vi "ReadCurrent.vi"(8 "error in (no error)":errorcluster, 11 "reference in":refnum<class "VdPhilipsMM-456.lvclass">) -> (0 "error out":errorcluster, 2 "Current":dbl, 3 "reference out":refnum<class "VdPhilipsMM-456.lvclass">)   [LabVIEW 2020, in "MulitMeters.lvlib" / "VdPhilipsMM-456.lvclass"]
uses:
  VdPhilipsMM-456.lvclass
  VdPhilipsMM-456.lvclass/VdPhilipsMM-456.ctl
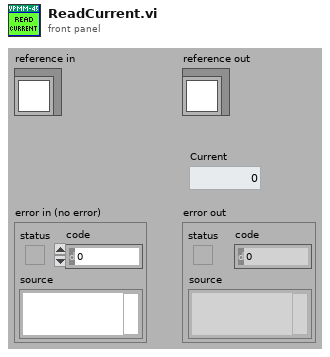
[diagram p1: front panel]
types:
  T1 = typedef "MulitMeters.lvlib/VdPhilipsMM-456.lvclass/ObjectAttributes.ctl" = cluster{"VISA Ref":refnum<visa-resource-name>}
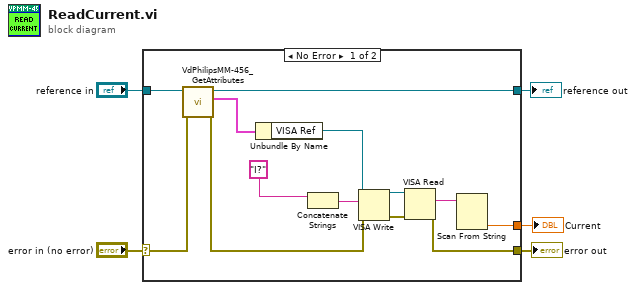
[diagram p0: block diagram]
diagram:
  n1 = case shown="No Error" "error in (no error)" {
    selector: "error in (no error)" -> [w18 w20]
    tunnel: [w9 w20] -> w4
    tunnel: [w15 w19] -> w2
    tunnel: "reference in" -> [w16 w19]
    tunnel: [w6 _] -> w1
    frame No Error {
      n2 = call "VdPhilipsMM-456_GetAttributes.vi"("error in (no error)"=w18, "reference in"=w16) -> ("error out"=w8:errorcluster, "Data"=w17:T1, "reference out"=w15:refnum<class "VdPhilipsMM-456.lvclass">)  [unwired: 6 in, 1 out]
      n3 = Unbundle By Name(w17) -> ("VISA Ref"=w14:refnum<visa-resource-name>)
      n4 = Concatenate Strings("I?") -> (w12:string)  [unwired: 1 in]
      n5 = VISA Write(VISA resource name=w14, write buffer=w12, error in (no error)=w8) -> (VISA resource name out=w10:refnum<visa-resource-name>, error out=w11:errorcluster)  [unwired: 1 out]
      n6 = VISA Read(VISA resource name=w10, error in (no error)=w11) -> (read buffer=w7:string, error out=w9:errorcluster)  [unwired: 1 in, 2 out]
      n7 = Scan From String(input string=w7) -> (output 1=w6:dbl)  [unwired: 4 in, 3 out]
    }
    frame Error {
    }
  }
  "error out" <- w4
  "reference out" <- w2
  "Current" <- w1
